vi "Unflatten-TextEditingCandidatesEventData.vi"(8 "error in (no error)":errorcluster, 11 "Event Binary Data":string) -> (0 "error out":errorcluster, 3 "Event Data":T1)   [LabVIEW 2026, in "SDL3.lvlib" / "Events.lvlib"]
uses:
  Events.lvlib
  Video/WindowID--integer.ctl
  Video/Video.lvlib
  TextEditingCandidatesEventData--cluster.ctl
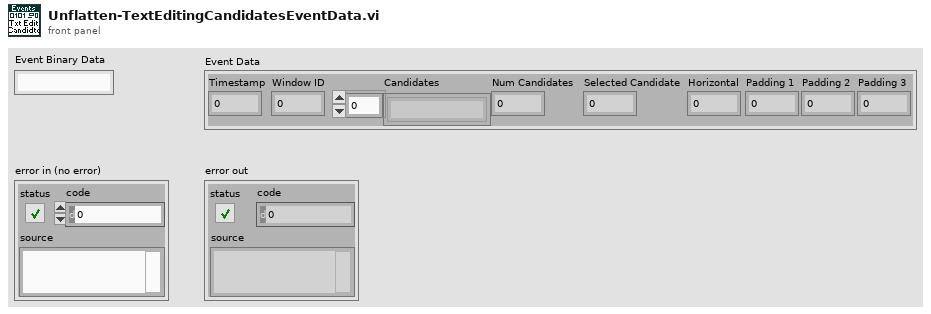
[diagram p1: front panel]
types:
  T1 = typedef "SDL3.lvlib/Events.lvlib/TextEditingCandidatesEventData--cluster.ctl" = cluster{"Timestamp":u64, "Window ID":T2, "Candidates":string[], "Num Candidates":i32, "Selected Candidate":i32, "Horizontal":i32, "Padding 1":u8, "Padding 2":u8, "Padding 3":u8}
  T2 = typedef "SDL3.lvlib/Video.lvlib/WindowID--integer.ctl" = u32
  T3 = enum16{"big-endian, network order", "native, host order", "little-endian"}
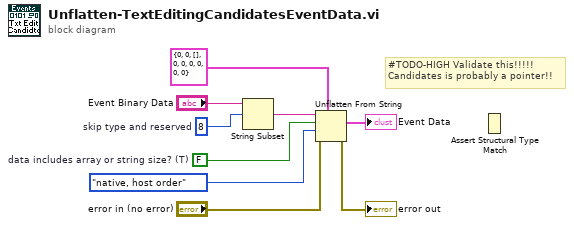
[diagram p0: block diagram]
diagram:
  w3 = 8  # skip type and reserved
  w6 = FALSE  # data includes array or string size? (T)
  # "#TODO-HIGH Validate this!!!!!\nCandidates is probably a pointer!!"
  n1 = String Subset(string="Event Binary Data", offset (0)=w3) -> (substring=w4:string)  [unwired: 1 in]
  n2 = Unflatten From String(type=T1 {"Timestamp"=0, "Window ID"=0, "Candidates"=[], "Num Candidates"=0, "Selected Candidate"=0, "Horizontal"=0, "Padding 1"=0, "Padding 2"=0, "Padding 3"=0} ("TextEditingEvent"), binary string=w4, data includes array or string size? (T)=w6, byte order (0:big-endian, network order)=T3."native, host order", error in (no error)="error in (no error)") -> (value=→"Event Data":T1, error out=→"error out":errorcluster)  [unwired: 1 out]
  n3 = Assert Structural Type Match() -> ()  [unwired: 2 in]
